vi "ReportError.vi"(0 "Convert to warning":bool, 5 "Error In":errorcluster) -> (19 "Error Out":errorcluster)   [LabVIEW 2019, in "Error handler.lvclass"]
uses:
  Error handler.lvclass
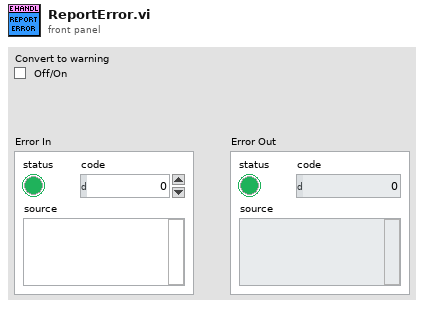
[diagram p1: front panel]
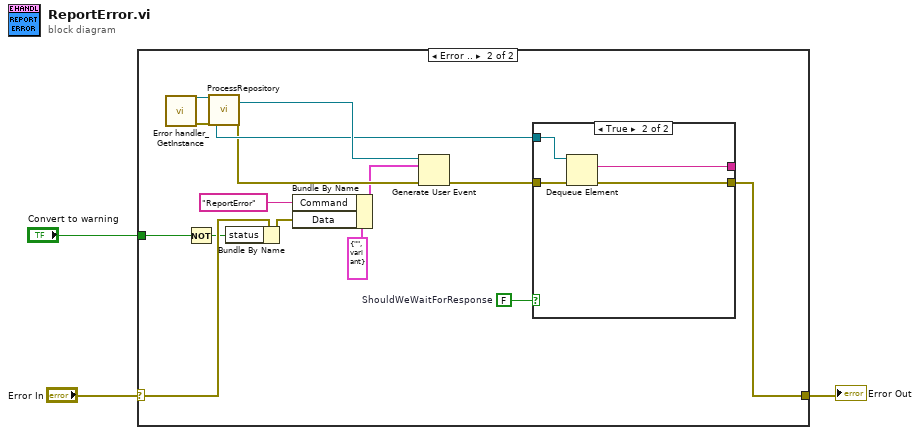
[diagram p0: block diagram]
diagram:
  n1 = case shown="Error .." "Error In" {
    selector: "Error In" -> [w4 w19]
    tunnel: [w4 w8] -> w2
    tunnel: "Convert to warning" -> [_ w6]
    frame No Error {
    }
    frame Error {
      w17 = FALSE  # ShouldWeWaitForResponse
      n2 = call "Error handler_GetInstance.vi"() -> ("reference out"=w13:refnum<class "Error handler.lvclass">, "error out"=w12:errorcluster)  [unwired: 15 in, 3 out]
      n3 = Not(x=w6) -> (.not. x?=w5:bool)
      n4 = call "ProcessRepository.vi"("reference in"=w13, "Error In"=w12) -> ("QueueFromProcess"=w15:refnum<queue>, "EventsToProcess"=w18:refnum<user-event>, "Error Out"=w14:errorcluster)  [unwired: 10 in, 5 out]
      n5 = Bundle By Name(cluster=w19, "status"=w5) -> (w7:errorcluster)
      n6 = Bundle By Name(cluster=cluster{"Command":string, "Data":variant} {"Command"="", "Data"=variant} ("MessageToProcess"), "Command"="ReportError", "Data"=w7) -> (w10:cluster{"Command":string, "Data":variant})
      n7 = Generate User Event(user event=w18, event data cluster=w10, error in=w14) -> (error out=w16:errorcluster)  [unwired: 1 in, 1 out]
      n8 = case shown="True" w17 {
        tunnel: w16 -> [w20 w24]
        tunnel: w15 -> [_ w23]
        tunnel: [_ w22] -> _
        tunnel: [w20 w21] -> w8
        frame False {
        }
        frame True {
          n9 = Dequeue Element(queue=w23, error in (no error)=w24) -> (element=w22:string, error out=w21:errorcluster)  [unwired: 1 in, 2 out]
        }
      }
    }
  }
  "Error Out" <- w2
